vi "GL_Pgain.vi"() -> ()   [LabVIEW 2024]
panel:
  out "P":dbl min=0.0 max=100.0 step=0.01 format="%.2f"
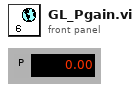
[diagram p1: front panel]
diagram:
